vi "mainFPGA.vi"() -> ()   [LabVIEW 2021]
uses:
  <vilib>/rvi/Emulation/niFpgaGetClockAttributes.vi
  <vilib>/rvi/Emulation/niFpgaSctlEmulationGetInTimedLoop.vi
  <vilib>/rvi/Emulation/niFpgaEmulationReportErrorSimple.vi
  <vilib>/rvi/eio/common/nirviEmuTemplateMethod_errors.vi
  <vilib>/rvi/Emulation/niFpgaCriticalErrorInLSC.vi
  <vilib>/rvi/interface/RandomDataEmulation/niFpgaRandomDataHandleErrors.vi
  <vilib>/eio/EIONode/EIONode.xnode
  <vilib>/rvi/DataTransferAndStorage/Container/XNode/niFpgaContainer.xnode
  <vilib>/rvi/interface/RandomDataEmulation/nirviRandomDataFpgaReadWriteTemplate.vi
panel:
  out "UserSwitches3:0":bool[](array[boolean])
  out "iterations_u8fifo":i32
  out "iterations_fifo_AB":i32
  out "User Switch3:0":u8
  in  "Wait (mSec)":u32=200
  out "UserSwitch0":bool
  out "UserSwitch1":bool
  in  "UserLED0":bool
  in  "UserLED1":bool
  in  "UserLED2":bool
  in  "UserLED3":bool
  out "User Switch2":bool
  out "UserSwitch3":bool
  out "iterations_loop_switches":i32
  out "FIFO_A Timed Out?":bool
  out "FIFO_B Timed Out?":bool
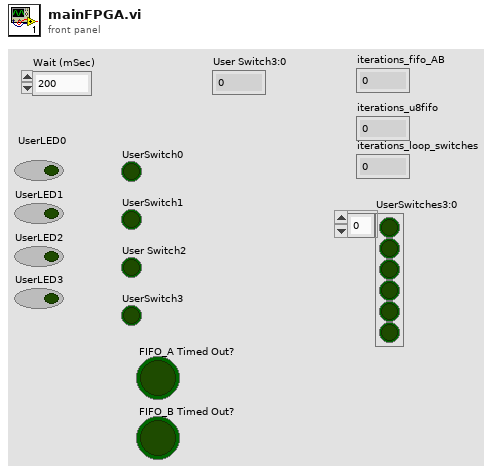
[diagram p1: front panel]
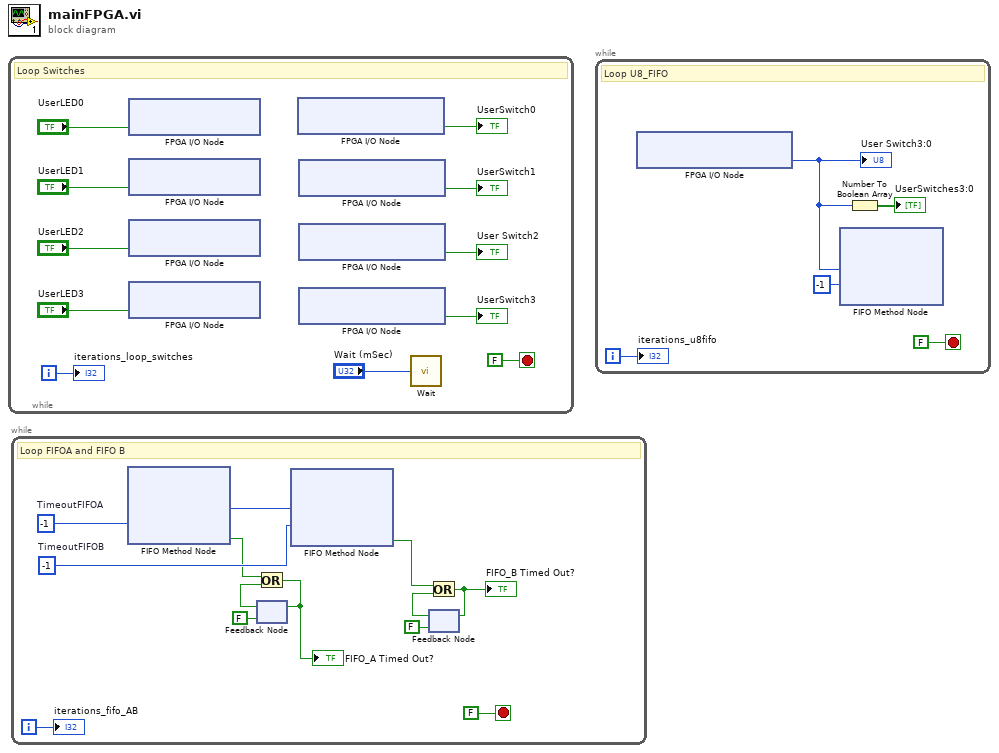
[diagram p0: block diagram]
diagram:
  n1 = while {
    i -> [w3]
    stop <- FALSE stop-if-true
    # "Loop Switches"
    n2 = xnode "FPGA I/O Node"("Mod1/User LED0"="UserLED0") -> ()  [unwired: 1 in, 1 out]
    n3 = xnode "FPGA I/O Node"("Mod1/User LED1"="UserLED1") -> ()  [unwired: 1 in, 1 out]
    n4 = xnode "FPGA I/O Node"("Mod1/User LED2"="UserLED2") -> ()  [unwired: 1 in, 1 out]
    n5 = xnode "FPGA I/O Node"("Mod1/User LED3"="UserLED3") -> ()  [unwired: 1 in, 1 out]
    n6 = xnode "FPGA I/O Node"() -> ("Mod1/User Switch0"=→"UserSwitch0":bool)  [unwired: 1 in, 1 out]
    n7 = xnode "FPGA I/O Node"() -> ("Mod1/User Switch1"=→"UserSwitch1":bool)  [unwired: 1 in, 1 out]
    n8 = xnode "FPGA I/O Node"() -> ("Mod1/User Switch2"=→"User Switch2":bool)  [unwired: 1 in, 1 out]
    n9 = xnode "FPGA I/O Node"() -> ("Mod1/User Switch3"=→"UserSwitch3":bool)  [unwired: 1 in, 1 out]
    n10 = call "Wait"("Count(mSec)"="Wait (mSec)") -> ()  [unwired: 1 out]
    "iterations_loop_switches" <- w3
  }
  n11 = while {
    i -> [w12]
    stop <- FALSE stop-if-true
    w23 = -1  # TimeoutFIFOB
    w22 = -1  # TimeoutFIFOA
    # "Loop FIFOA and FIFO B"
    n12 = xnode ("FIFO Method Node")("Timeout"=w22) -> ("Element"=w24:i16, "Timed Out?"=w18:bool)  [unwired: 2 in, 2 out]
    n13 = feedback #1(FALSE) -> (w20:bool)
    n14 = Or(x=w18, y=w20) -> (x .or. y?=w14:bool)
    "FIFO_A Timed Out?" <- w14
    n15 = feedback-in #1(w14) -> ()
    n16 = xnode ("FIFO Method Node")("Element"=w24, "Timeout"=w23) -> ("Timed Out?"=w15:bool)  [unwired: 2 in, 2 out]
    n17 = feedback #2(FALSE) -> (w16:bool)
    n18 = Or(x=w15, y=w16) -> (x .or. y?=w13:bool)
    "FIFO_B Timed Out?" <- w13
    n19 = feedback-in #2(w13) -> ()
    "iterations_fifo_AB" <- w12
  }
  n20 = while {
    i -> [w28]
    stop <- FALSE stop-if-true
    # "Loop U8_FIFO"
    n21 = xnode "FPGA I/O Node"() -> ("Mod1/User Switch3:0"=w26:u8)  [unwired: 1 in, 1 out]
    "User Switch3:0" <- w26
    n22 = xnode ("FIFO Method Node")("Element"=w26, "Timeout"=-1) -> ()  [unwired: 1 in, 2 out]
    n23 = Number To Boolean Array(number=w26) -> (Boolean array=→"UserSwitches3:0":bool[])
    "iterations_u8fifo" <- w28
  }
